vi "Audiogram-Read File.vi"(0 "Audiogram File":path, 11 "error in":errorcluster) -> (3 "MinPowerFreq (Hz)":dbl, 4 "Freq (Hz)":dbl[](array[numeric]), 6 "Magnitude (dB)":dbl[](array[numeric]), 8 "MinFreq (Hz)":dbl, 10 "MaxFreq (Hz)":dbl, 14 "Min Threshold (dB SPL)":dbl, 15 "error out":errorcluster)   [LabVIEW 2020]
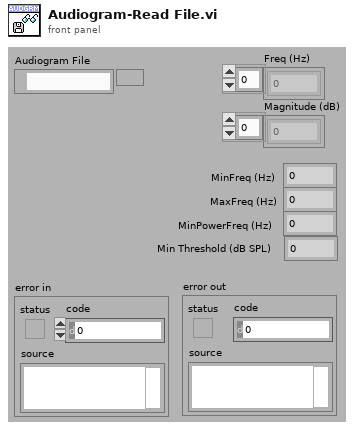
[diagram p1: front panel]
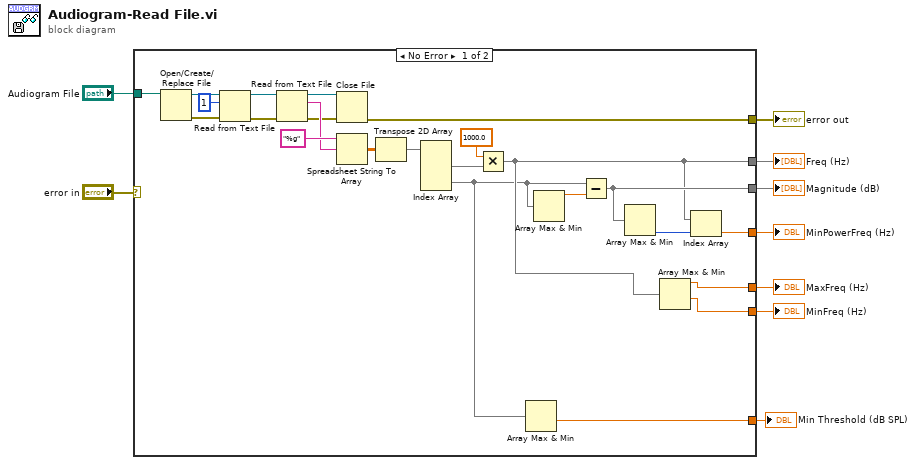
[diagram p0: block diagram]
diagram:
  n1 = case shown="No Error" "error in" {
    selector: "error in" -> [_ w34]
    tunnel: [w10 _] -> w9
    tunnel: [w11 _] -> w8
    tunnel: [w14 _] -> w7
    tunnel: [w17 _] -> w6
    tunnel: [w31 w34] -> w5
    tunnel: "Audiogram File" -> [w19 _]
    tunnel: [w16 _] -> w2
    tunnel: [w12 _] -> w1
    frame No Error {
      n2 = Open/Create/Replace File(file path (use dialog)=w19) -> (refnum out=w21:refnum<file>, error out=w20:errorcluster)  [unwired: 5 in, 1 out]
      n3 = Read from Text File(file (use dialog)=w21, count=1, error in=w20) -> (refnum out=w24:refnum<file>, error out=w23:errorcluster)  [unwired: 1 in, 2 out]
      n4 = Read from Text File(file (use dialog)=w24, error in=w23) -> (refnum out=w26:refnum<file>, text=w27:string, error out=w25:errorcluster)  [unwired: 2 in, 1 out]
      n5 = Close File(refnum=w26, error in=w25) -> (error out=w31:errorcluster)  [unwired: 1 out]
      n6 = Spreadsheet String To Array(format string="%g", spreadsheet string=w27) -> (array=w29:dbl[][])  [unwired: 2 in]
      n7 = Transpose 2D Array(2D array=w29) -> (transposed array=w30:dbl[][])
      n8 = Index Array(array=w30) -> (element #1=w32:dbl[], element #2=w13:dbl[])  [unwired: 4 in]
      n9 = Multiply(x=1000.0, y=w32) -> (x*y=w14:dbl[])
      n10 = Array Max & Min(array=w13) -> (min value=w12:dbl)  [unwired: 3 out]
      n11 = Array Max & Min(array=w13) -> (max value=w18:dbl)  [unwired: 3 out]
      n12 = Subtract(x=w13, y=w18) -> (x-y=w17:dbl[])
      n13 = Array Max & Min(array=w17) -> (min index (indices)=w15:i32)  [unwired: 3 out]
      n14 = Array Max & Min(array=w14) -> (max value=w10:dbl, min value=w11:dbl)  [unwired: 2 out]
      n15 = Index Array(array=w14, index=w15) -> (element=w16:dbl)
    }
    frame Error {
    }
  }
  "MaxFreq (Hz)" <- w9
  "MinFreq (Hz)" <- w8
  "Freq (Hz)" <- w7
  "Magnitude (dB)" <- w6
  "error out" <- w5
  "MinPowerFreq (Hz)" <- w2
  "Min Threshold (dB SPL)" <- w1
